vi "from string.vi"(8 "error in":errorcluster, 9 "channel data":string, 10 "identifier":string, 11 "channel in":refnum<class "fifo channel.lvclass">) -> (0 "error out":errorcluster, 3 "channel out":refnum<class "fifo channel.lvclass">)   [LabVIEW 2014, in "fifo channel.lvclass"]
uses:
  fifo channel.lvclass
  fifo channel.lvclass/fifo channel.ctl
  Read fifo config.vi
  Write fifo config.vi
  <vilib>/NI/Tag Bus Module Framework/channel/TBM channel.lvclass
  <vilib>/NI/Configuration Framework/serializable configuration/NISE_CEF_serializable configuration.lvclass
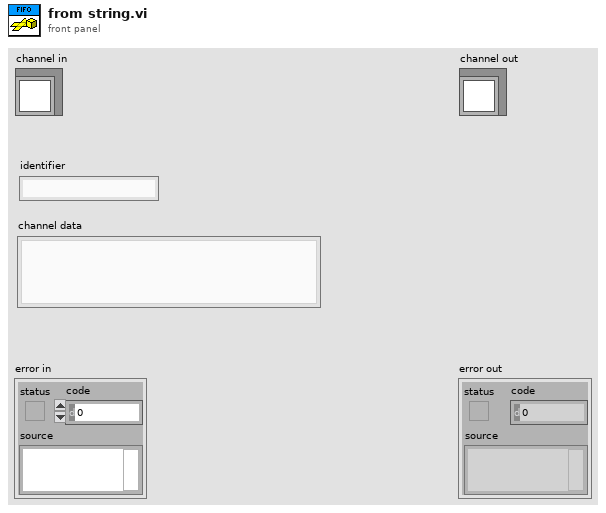
[diagram p1: front panel]
types:
  T1 = typedef "fifo channel.lvclass/fifo channel settings.ctl" = cluster{"Timeout":string, "Reset":string, "Averages":i32, "Samples":u32, "Channels":i32, "Fifo size":u32}
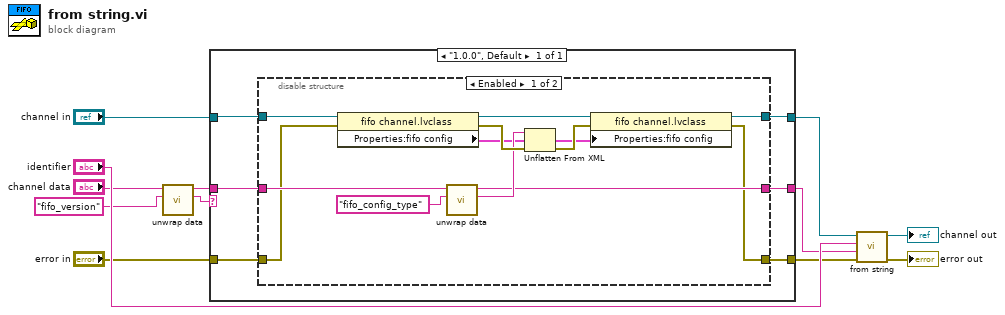
[diagram p0: block diagram]
diagram:
  n1 = call <vilib>:"unwrap data.vi"("identifier"="fifo_version", "data to unwrap"="channel data") -> ("unwrapped data"=w10:string, "remaining string"=w9:string)  [unwired: 8 in]
  n2 = case shown="\"1.0.0\", Default" w10 {
    tunnel: "error in" -> [w15]
    tunnel: w9 -> [w17]
    tunnel: "channel in" -> [w14]
    tunnel: [w18] -> w7
    tunnel: [w16] -> w5
    tunnel: [w13] -> w4
    frame "1.0.0", Default {
      n3 = disable-structure shown="Enabled" {
        disable-tunnel: [w29 w34] -> w18
        disable-tunnel: w17 -> [w28 w33]
        disable-tunnel: [w25 w33] -> w16
        disable-tunnel: w15 -> [w22 w32]
        disable-tunnel: w14 -> [w21 w34]
        disable-tunnel: [w19 w32] -> w13
        frame Enabled {
          n4 = property class="fifo channel.lvclass"(reference=w21, error in=w22) -> (reference out=w20:refnum<class "fifo channel.lvclass">, error out=w31:errorcluster, "Properties:fifo config"=w23:T1)
          n5 = call <vilib>:"unwrap data.vi"("identifier"="fifo_config_type" ("additional identifier"), "data to unwrap"=w28) -> ("unwrapped data"=w26:string, "remaining string"=w25:string)  [unwired: 8 in]
          n6 = Unflatten From XML(xml string=w26, type=w23, error in (no error)=w31) -> (value=w24:T1, error out=w30:errorcluster)
          n7 = property class="fifo channel.lvclass"(reference=w20, error in=w30, "Properties:fifo config"=w24) -> (reference out=w29:refnum<class "fifo channel.lvclass">, error out=w19:errorcluster)
        }
        frame Disabled {
        }
      }
    }
  }
  n8 = call-parent "from string.vi"("error in"=w4, "channel data"=w5, "identifier"="identifier", "channel in"=w7) -> ("error out"=→"error out":errorcluster, "channel out"=→"channel out":refnum<class "fifo channel.lvclass">)  [unwired: 6 in]
